vi "Gui_SetupTimingTable.vi"(0 "QMH UI References.Refnum TIMING Table":refnum<vi>, 3 "error in (no error)":errorcluster) -> (7 "QMH UI References.Refnum TIMING Table Output":refnum<vi>, 10 "error out":errorcluster caption="sortie d'erreur")   [LabVIEW 2018]
doc: "This VI setup the TIMING Table parameters.\n\n1. The TIMING Table parameters are passed by a reference of the QMH UI References pool.\n2. Fill the control TIMING Table with last values\n3. Wait for the user events, and update controls accordingly.\n4. When OK is pushed, return the reference to the updated values of Timing Table"
uses:
  controls/TIMING_Table.ctl
  controls/TIMING_Mandatory_Items.ctl
  controls/TIMING_Optional_Items.ctl
panel:
  in  "TIMING Table":T1={"Mandatory Items"={"Script Name"="", "HSDIO Delay"=60.0, "Shutter Duration before"=50000.0, "Shutter Duration after"=50000.0, "Filter Tau"=2.0, "Trapping Delay"=600.0, "Trapping Duration"=300.0, "Emtyping Duration"=1000.0}, "Optional Items"={"Eject"=0, "Acq"=0, "Excit"=0, "Gas"=0, "Laser"=0, "Lamp"=0}, "Times Table"=[["Excit1", "name", "Swift", "0.5", "1200", "70", "150", "550", "0", "0", "0"]]} {"Optional Items"."Laser" min=0 max=3; "Optional Items"."Gas" min=0 max=5; "Mandatory Items"."Shutter Duration after" min=2.0 max=100000.0; "Mandatory Items"."HSDIO Delay" min=60.0 max=100.0; "Mandatory Items"."Shutter Duration before" min=2.0 max=100000.0; "Mandatory Items"."Filter Tau" min=1000.0 max=2000.0; "Mandatory Items"."Trapping Delay" min=2.0; "Mandatory Items"."Emtyping Duration" min=2.0 format="%#_8g"; "Mandatory Items"."Trapping Duration" min=2.0}
  in  "OK":bool
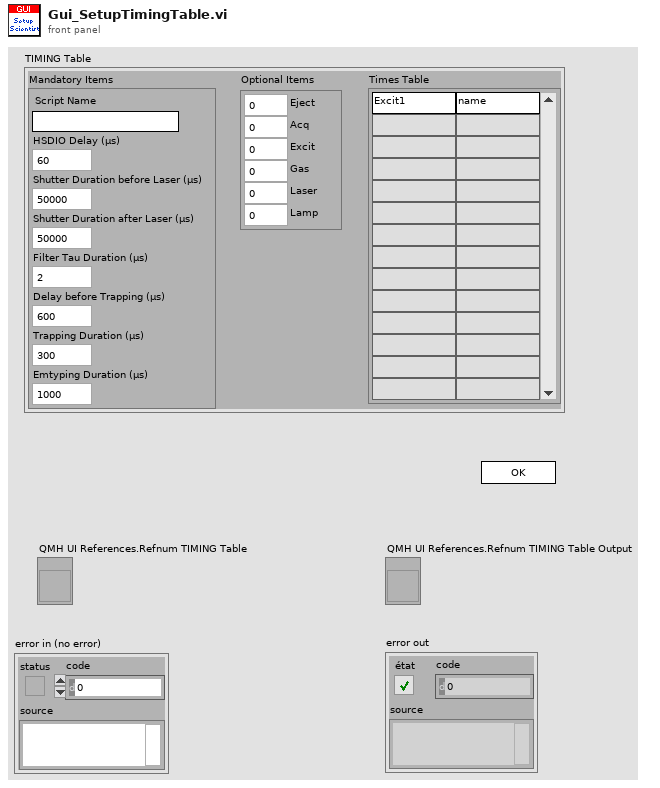
[diagram p1: front panel]
types:
  T1 = typedef "TIMING_Table.ctl" = cluster{"Mandatory Items":T2, "Optional Items":T3, "Times Table":string[][]}
  T2 = typedef "TIMING_Mandatory_Items.ctl" = cluster{"Script Name":string, "HSDIO Delay":dbl, "Shutter Duration before":dbl, "Shutter Duration after":dbl, "Filter Tau":dbl, "Trapping Delay":dbl, "Trapping Duration":dbl, "Emtyping Duration":dbl}
  T3 = typedef "TIMING_Optional_Items.ctl" = cluster{"Eject":u32, "Acq":i32, "Excit":u32, "Gas":i32, "Laser":i32, "Lamp":i32}
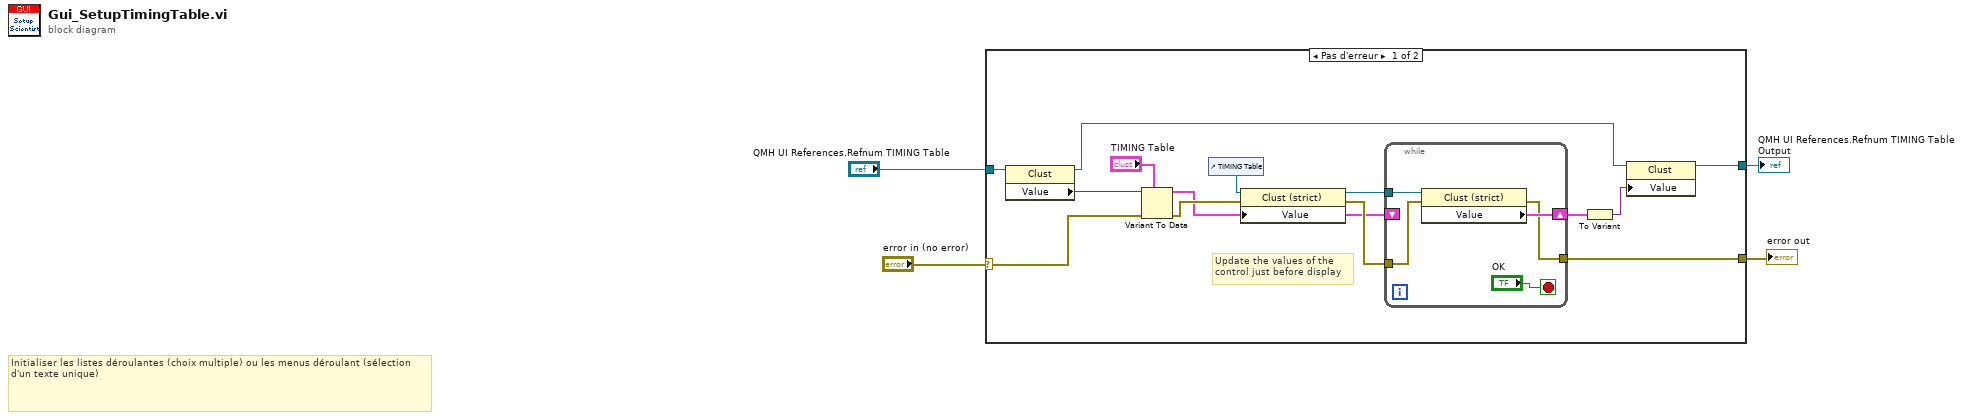
[diagram p0: block diagram]
diagram:
  # "Initialiser les listes déroulantes (choix multiple) ou les menus déroulant (sélection d'un texte unique)"
  n1 = case shown="Pas d'erreur" "error in (no error)" {
    selector: "error in (no error)" -> [w18 w25]
    tunnel: [w14 w25] -> w4
    tunnel: "QMH UI References.Refnum TIMING Table" -> [w13 w24]
    tunnel: [w6 w24] -> w1
    frame No Error {
      # "Update the values of the\ncontrol just before display"
      n2 = property class="Clust"(reference=w13) -> (reference out=w7:refnum<vi>, "Value"=w12:variant)  [unwired: 1 in, 1 out]
      n3 = Variant To Data(error in=w18, type="TIMING Table", Variant=w12) -> (data=w11:T1, error out=w17:errorcluster)
      n4 = control-ref of="TIMING Table"() -> (w10:refnum<vi>)
      n5 = property class="Clust (strict)"(reference=w10, error in=w17, "Value"=w11) -> (reference out=w15:refnum<vi>, error out=w16:errorcluster)
      n6 = while {
        shift-right: [w21] -> w9
        shift-left: w11 -> [_]
        tunnel: w16 -> [w20]
        tunnel: w15 -> [w22]
        tunnel: [w19] -> w14
        stop <- "OK" stop-if-true
        n7 = property class="Clust (strict)"(reference=w22, error in=w20) -> (error out=w19:errorcluster, "Value"=w21:T1)  [unwired: 1 out]
      }
      n8 = To Variant(anything=w9) -> (Variant=w8:variant)
      n9 = property class="Clust"(reference=w7, "Value"=w8) -> (reference out=w6:refnum<vi>)  [unwired: 1 in, 1 out]
    }
    frame Error {
    }
  }
  "error out" <- w4
  "QMH UI References.Refnum TIMING Table Output" <- w1
